vi "Convert Channel Settings to Digital.vi"(11 "channel settings":T1[](array[typedef])) -> (2 "channel default values":dbl[](array[numeric]), 3 "channel names":string[](array[string]))   [LabVIEW 2020, in "Scan Engine Scripting.lvlib"]
uses:
  Scan Engine Scripting.lvlib
  Modules/Mode Classes/Controls/digital channel settings.ctl
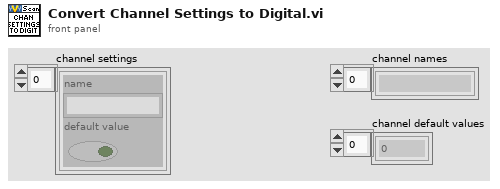
[diagram p1: front panel]
types:
  T1 = typedef "Scan Engine Scripting.lvlib/digital channel settings.ctl" = cluster{"name":string, "default value":bool}
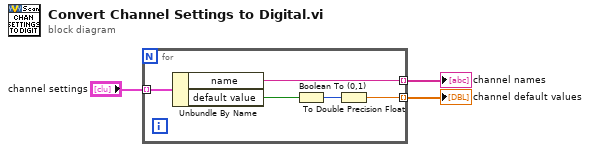
[diagram p0: block diagram]
diagram:
  n1 = for {
    tunnel: "channel settings" -> [w8] mode=indexing
    tunnel: [w7] -> w2 mode=indexing
    tunnel: [w4] -> w3 mode=indexing
    n2 = Unbundle By Name(w8) -> ("name"=w7:string, "default value"=w5:bool)
    n3 = Boolean To (0,1)(Boolean=w5) -> (0, 1=w6:i16)
    n4 = To Double Precision Float(number=w6) -> (double precision float=w4:dbl)
  }
  "channel default values" <- w3
  "channel names" <- w2
